vi "EIP channel to string.vi"(11 "channel in":refnum<class "EthernetIP Channel.lvclass">) -> (2 "channel data":string, 3 "identifier":string)   [LabVIEW 2013, in "EthernetIP Channel.lvclass"]
uses:
  EthernetIP Channel.lvclass
  <vilib>/NI/Tag Bus/tag/tag descriptor.lvclass/tag descriptor.ctl
  <vilib>/NI/Tag Bus Module Framework/channel/TBM channel.lvclass/TBM channel.ctl
  EthernetIP Channel.lvclass/EthernetIP Channel.ctl
  <vilib>/NI/Tag Bus/tag/tag descriptor.lvclass
  <vilib>/NI/Tag Bus Module Framework/channel/TBM channel.lvclass
  <vilib>/NI/Configuration Framework/serializable configuration/NISE_CEF_serializable configuration.lvclass
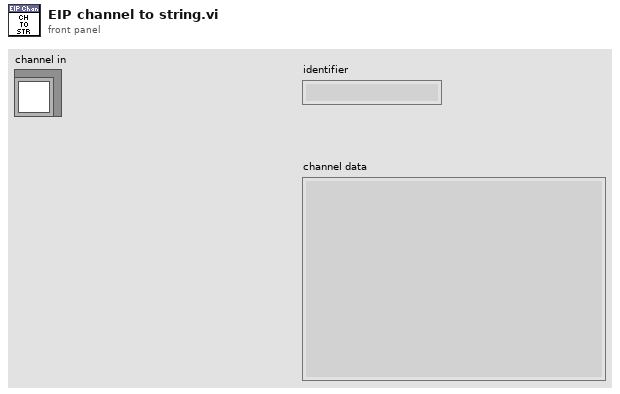
[diagram p1: front panel]
types:
  T1 = typedef "tag bus.lvlib/tag descriptor.lvclass/Data Type.ctl" = enum16{"Double", "Single", "I64", "I32", "I16", "I8", "U64", "U32", "U16", "U8", "Boolean", "String", "Array of Double", "Array of Single", "Array of I64", "Array of I32", "Array of I16", "Array of I8", "Array of U64", "Array of U32", "Array of U16", "Array of U8", "Array of Boolean", "Array of String"}
  T2 = typedef "TBM channel.lvclass/channel classification.ctl" = enum16{"input data", "output data", "processing parameter", "processing result"}
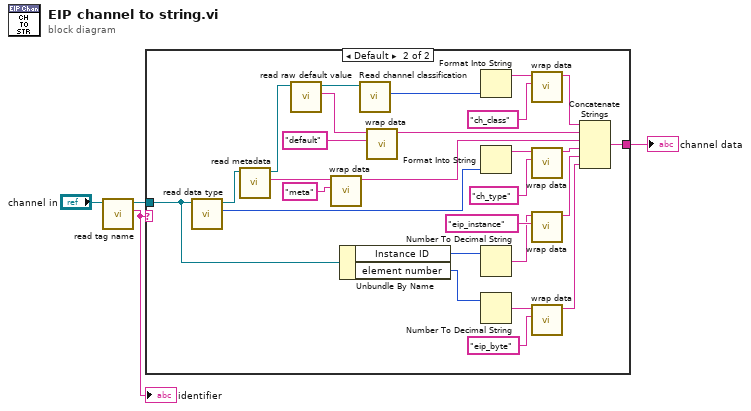
[diagram p0: block diagram]
diagram:
  n1 = call <vilib>:"read tag name.vi"("system tag in"="channel in") -> ("name"=w1:string, "system tag out"=w2:refnum<class "EthernetIP Channel.lvclass">)  [unwired: 8 in, 1 out]
  "identifier" <- w1
  n2 = case shown="Default" w1 {
    selector: w1 -> [w5 _]
    tunnel: [w5 w15] -> w4
    tunnel: w2 -> [_ w14]
    frame "" {
    }
    frame Default {
      n3 = call <vilib>:"read data type.vi"("system tag in"=w14) -> ("data type"=w30:T1, "system tag out"=w32:refnum<class "EthernetIP Channel.lvclass">)  [unwired: 8 in, 1 out]
      n4 = call <vilib>:"read metadata.vi"("system tag in"=w32) -> ("metadata"=w25:string, "system tag out"=w31:refnum<class "EthernetIP Channel.lvclass">)  [unwired: 8 in, 1 out]
      n5 = call <vilib>:"read raw default value.vi"("system tag in"=w31) -> ("raw default"=w24:string, "system tag out"=w27:refnum<class "EthernetIP Channel.lvclass">)  [unwired: 8 in, 1 out]
      n6 = call <vilib>:"wrap data.vi"("identifier"="meta", "data to wrap"=w25) -> ("wrapped data"=w17:string)  [unwired: 9 in]
      n7 = Unbundle By Name(w14) -> ("Instance ID"=w12:u32, "element number"=w13:i32)
      n8 = call <vilib>:"Read channel classification.vi"("channel in"=w27) -> ("channel classification"=w22:T2)  [unwired: 8 in, 2 out]
      n9 = call <vilib>:"wrap data.vi"("identifier"="default", "data to wrap"=w24) -> ("wrapped data"=w18:string)  [unwired: 9 in]
      n10 = Format Into String(w22) -> (resulting string=w21:string)  [unwired: 3 in, 1 out]
      n11 = Format Into String(w30) -> (resulting string=w29:string)  [unwired: 3 in, 1 out]
      n12 = Number To Decimal String(number=w12) -> (decimal integer string=w8:string)  [unwired: 1 in]
      n13 = Number To Decimal String(number=w13) -> (decimal integer string=w9:string)  [unwired: 1 in]
      n14 = call <vilib>:"wrap data.vi"("identifier"="ch_class", "data to wrap"=w21) -> ("wrapped data"=w19:string)  [unwired: 9 in]
      n15 = call <vilib>:"wrap data.vi"("identifier"="ch_type", "data to wrap"=w29) -> ("wrapped data"=w16:string)  [unwired: 9 in]
      n16 = call <vilib>:"wrap data.vi"("identifier"="eip_instance", "data to wrap"=w8) -> ("wrapped data"=w6:string)  [unwired: 9 in]
      n17 = call <vilib>:"wrap data.vi"("identifier"="eip_byte", "data to wrap"=w9) -> ("wrapped data"=w7:string)  [unwired: 9 in]
      n18 = Concatenate Strings(w19, w18, w17, w16, w6, w7) -> (w15:string)
    }
  }
  "channel data" <- w4
